vi "sub_temperature-n.vi"(9 "n":i32, 10 "Channel":u16(ring)=3 items=["", "CH1", "CH2", "CH3", "CH4", "CH5", "CH6", "CH7", "CH8", "CH9", "CH10", "CH11", "CH12", "CH13", "CH14", "CH15", "CH16"], 11 "visa":refnum<visa-resource-name>) -> (3 "temp chart":dbl(graph))   [LabVIEW 2019]
uses:
  44da94d6-71ab-4a60-8969-1b02bc56d179.vi
  <instrlib>/Yokogawa DL950 Series/Public/Configure/Configure Module (Temperature).vi
  <instrlib>/Yokogawa DL950 Series/Yokogawa DL950 Series.lvlib
panel:
  out "temp Value":dbl format="%.3p"
  out "time":u32
  out "error out":errorcluster
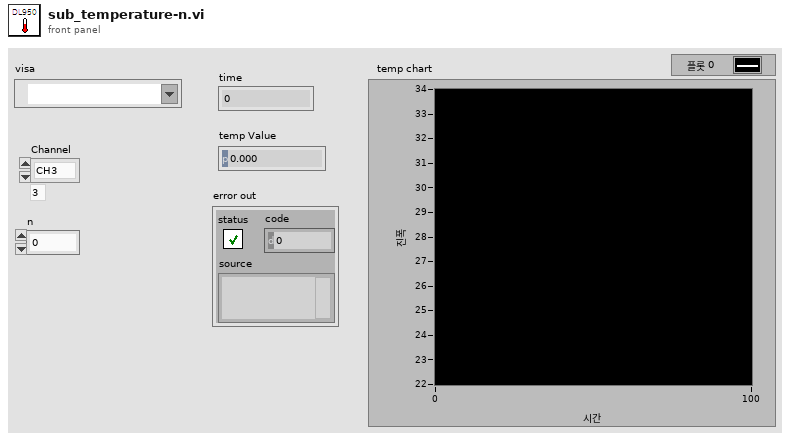
[diagram p1: front panel]
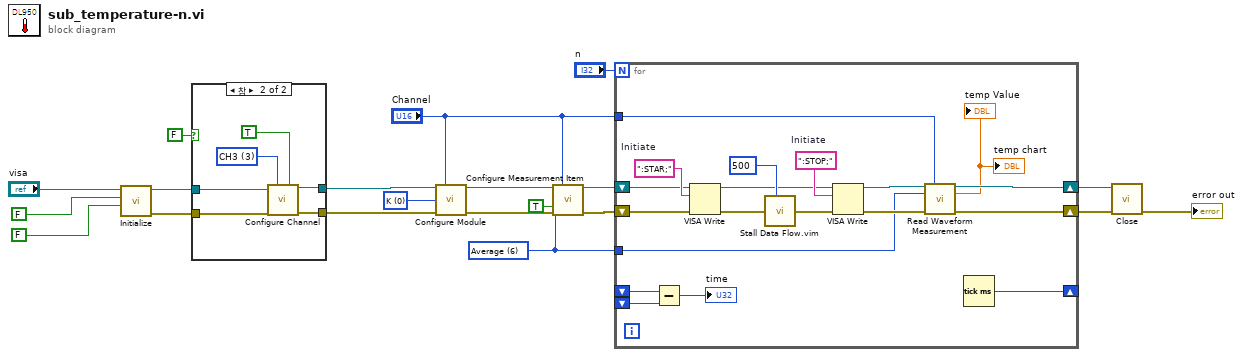
[diagram p0: block diagram]
diagram:
  w4 = 6 items=["Peak to Peak", "Amplitude", "Max", "Min", "High", "Low", "Average", "Middle", "Rms", "Standard Deviation", "+Overshoot", "-Overshoot", "Rise", "Fall", "Frequency", "Period", "+Width", "-Width", "Duty Cycle", "Pulse Count", "Burst1 Width", "Burst2 Width", "Average Frequency", "Average Period", "Int1TY", "Int2TY"] ("Measurement Item (0: Peak to Peak)")
  w16 = 0 items=["K", "E", "J", "T", "L", "U", "N", "R", "S", "B", "W", "Au7fe"] ("Thermocouple Type (0: K)")
  n1 = call <instrlib>:"Initialize.vi"("Reset (True)"=FALSE, "ID Query (True)"=FALSE, "VISA resource name"="visa") -> ("error out"=w11:errorcluster, "VISA resource name out"=w13:refnum<visa-resource-name>)  [unwired: 7 in]
  n2 = case shown="참" FALSE {
    tunnel: w13 -> [w22 w28]
    tunnel: [w22 w27] -> w12
    tunnel: w11 -> [w21 w26]
    tunnel: [w21 w25] -> w10
    frame False {
    }
    frame True {
      w24 = u16 3 items=["", "CH1", "CH2", "CH3", "CH4", "CH5", "CH6", "CH7", "CH8", "CH9", "CH10", "CH11", "CH12", "CH13", "CH14", "CH15", "CH16", "RMATH1", "RMATH2", "RMATH3", "RMATH4", "RMATH5", "RMATH6", "RMATH7", "RMATH8", "RMATH9", "RMATH10", "RMATH11", "RMATH12", "RMATH13", "RMATH14", "RMATH15", "RMATH16"] ("Channel (1: CH1)")
      n3 = call <instrlib>:"Configure Channel.vi"("VISA resource name"=w28, "Channel (1: CH1)"=w24, "Enable Channel (True)"=TRUE, "error in (no error)"=w26) -> ("VISA resource name out"=w27:refnum<visa-resource-name>, "error out"=w25:errorcluster)  [unwired: 10 in]
    }
  }
  n4 = call-poly <instrlib>:"Configure Module.vi"("VISA resource name"=w12, "Channel (1: CH1)"="Channel", "Thermocouple Type (0: K)"=w16, "error in (no error)"=w10) -> ("VISA resource name out"=w9:refnum<visa-resource-name>, "error out"=w7:errorcluster)  [unwired: 10 in]
  n5 = call <instrlib>:"Configure Measurement Item.vi"("VISA resource name"=w9, "Source (1: CH1)"="Channel", "Measurement Item (0: Peak to Peak)"=w4, "Enable Measurement Item (False)"=TRUE, "error in (no error)"=w7) -> ("VISA resource name out"=w8:refnum<visa-resource-name>, "error out"=w6:errorcluster)  [unwired: 9 in]
  n6 = for {
    N: "n" -> [_]
    shift-right: [w33] -> w15
    shift-left: w8 -> [w42]
    shift-right: [w32] -> w14
    shift-left: w6 -> [w41]
    shift-right: [w47] -> _
    shift-left: _ -> [w46]
    shift-left: _ -> [w45]
    tunnel: w4 -> [w31]
    tunnel: "Channel" -> [w29]
    w40 = ":STOP;"  # Initiate
    w43 = ":STAR;"  # Initiate
    n7 = Subtract(x=w46, y=w45) -> (x-y=→"time":u32)
    n8 = VISA Write ("VISA書き込み")(VISA resource name=w42, write buffer=w43, error in (no error)=w41) -> (VISA resource name out=w36:refnum<visa-resource-name>, error out=w39:errorcluster)  [unwired: 1 out]
    n9 = call "Stall Data Flow.vim"("value in"=w39, "milliseconds to wait"=u32 500 ("dt")) -> ("value out"=w38:errorcluster)  [unwired: 1 out]
    n10 = VISA Write ("VISA書き込み")(VISA resource name=w36, write buffer=w40, error in (no error)=w38) -> (VISA resource name out=w35:refnum<visa-resource-name>, error out=w34:errorcluster)  [unwired: 1 out]
    n11 = call <instrlib>:"Read Waveform Measurement.vi"("VISA resource name"=w35, "Source (1: CH1)"=w29, "Measurement Item (0: Peak to Peak)"=w31, "error in (no error)"=w34) -> ("VISA resource name out"=w33:refnum<visa-resource-name>, "Measurement Value"=→"temp Value" →"temp chart":dbl, "error out"=w32:errorcluster)  [unwired: 9 in]
    n12 = Tick Count (ms)() -> (millisecond timer value=w47:u32)
  }
  n13 = call <instrlib>:"Close.vi"("error in (no error)"=w14, "VISA resource name"=w15) -> ("error out"=→"error out":errorcluster)  [unwired: 9 in]
